vi "WSVCAP SHL FPGA LL I2C Procedure - Send Data Byte.vi"(0 "Procedure Step":T1, 1 "Wait Ticks Remaining":u32, 5 "I2C Wait Ticks":u32, 7 "Write Bits Remaining":u8, 11 "error in (no error)":errorcluster, 13 "Socket Mask":u32 format="%06x", 14 "UUT (0/1)":u8) -> (3 "Wait Ticks Remaining Out":u32, 4 "Procedure Step Out":T1, 8 "Write Bits Remaining Out":u8, 10 "Finished":bool, 15 "error out":errorcluster)   [LabVIEW 2017]
uses:
  Type Defs/WSVCAP SHL Procedure Step Enum.ctl
  Type Defs/WSVCAP SHL FIFO Operation Enum.ctl
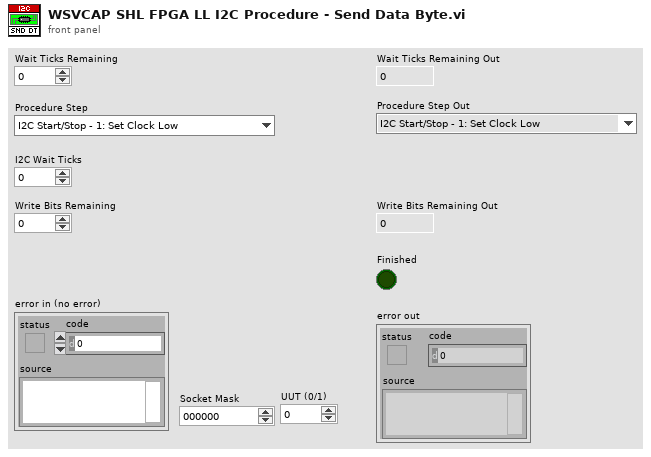
[diagram p1: front panel]
types:
  T1 = typedef "WSVCAP SHL Procedure Step Enum.ctl" = enum16{"I2C Start/Stop - 1: Set Clock Low", "I2C Start/Stop - 2: Wait", "I2C Start/Stop - 3: Set Data I", "I2C Start/Stop - 4: Wait", "I2C Start/Stop - 5: Set Clock High", "I2C Start/Stop - 6: Wait", "I2C Start/Stop - 7: Set Data II", "I2C Start/Stop - 8: Wait", "I2C Start/Stop - 9: Set Clock Low", "I2C Start/Stop - 10: Wait", "I2C Read ACK - 1: Set Clock High", "I2C Read ACK - 2: Wait", "I2C Read ACK - 3: Read ACK Bit", "I2C Read ACK - 4: Wait", "I2C Read ACK - 5: Set Clock Low", "I2C Read ACK - 6: Wait", "I2C Write ACK - 1: Write ACK Bit", "I2C Write ACK - 2: Wait", "I2C Write ACK - 3: Set Clock High", "I2C Write ACK - 4: Wait", "I2C Write ACK - 5: Set Clock Low", "I2C Write ACK - 6: Wait", "I2C Write ACK - 7: Set Data Low", "I2C Send Add - 1: Reset Bits Remaining", "I2C Send Add - 2: Set Data Bit", "I2C Send Add - 3: Wait", "I2C Send Add - 4: Set Clock High", "I2C Send Add - 5: Wait", "I2C Send Add - 6: Set Clock Low", "I2C Send Add - 7: Wait", "I2C Send Add - 8: Check Bits Remaining", "I2C Send Data - 1: Reset Bits Remaining", "I2C Send Data - 2: Load Write Bit from FIFO", "I2C Send Data - 3: Set Data Bit", "I2C Send Data - 4: Wait", "I2C Send Data - 5: Set Clock High", "I2C Send Data - 6: Wait", "I2C Send Data - 7: Set Clock Low", "I2C Send Data - 8: Wait", "I2C Send Data - 9: Check Bits Remaining", "I2C Receive Data - 1: Reset Bits Remaining", "I2C Receive Data - 2: Wait", "I2C Receive Data - 3: Set Clock High", "I2C Receive Data - 4: Wait", "I2C Receive Data - 5: Read Data Bit", "I2C Receive Data - 6: Wait", "I2C Receive Data - 7: Set Clock Low", "I2C Receive Data - 8: Wait", "I2C Receive Data - 9: Check Bits Remaining", "RFFE Send SSC - 1:Set Low", "RFFE Send SSC - 2:Wait", "RFFE Send SSC - 3:Set SDA High", "RFFE Send SSC - 4:Wait", "RFFE Send SSC - 5:Set SDA Low", "RFFE Send SSC - 6:Wait", "RFFE Send Data - 1:Set SCL High", "RFFE Send Data - 2:Wait", "RFFE Send Data - 3:Set SCL Low", "RFFE Send Data - 4:Wait", "RFFE Send Data - 5:Set SCL High (P)", "RFFE Send Data - 6:Wait", "RFFE Send Data - 7:Set SCL Low (P)", "RFFE Send Data - 8:Wait", "RFFE Send Data - 9:Set SCL High (BP)", "RFFE Send Data - 10:Wait", "RFFE Send Data - 11:Set SCL Low (BP)", "RFFE Send Data - 12:Wait", "RFFE Receive Data - 1:Set SCL High", "RFFE Receive Data - 2:Wait", "RFFE Receive Data - 3:Set SCL Low", "RFFE Receive Data - 4:Wait", "RFFE Receive Data - 5:Set SCL High (BP)", "RFFE Receive Data - 6:Wait", "RFFE Receive Data - 7:Set SCL Low (BP)", "RFFE Receive Data - 8:Wait", "RFFE Wait CMD Delay - 1:Wait", "RFFE Clear Lines - 1:Clear", "SRL Write Data - 1:Set SYNC High", "SRL Write Data - 2:Wait SYNC Delay", "SRL Write Data - 3:Set SYNC Low", "SRL Write Data - 4:Set SCLK High", "SRL Write Data - 5:Wait", "SRL Write Data - 6:Set SCLK Low", "SRL Write Data - 7:Wait", "SRL Write Data - 8:Set SYNC High", "SRL Wait CMD Delay - 1:Wait", "SRL Clear Lines - 1:Clear"}
  T2 = typedef "WSVCAP SHL FIFO Operation Enum.ctl" = enum16{"Create FIFO/Memory", "Get Write FIFO Status", "Get Read FIFO Status", "Put Element in Write", "Put Element in Read", "Get Element from Write", "Get Element from Read"}
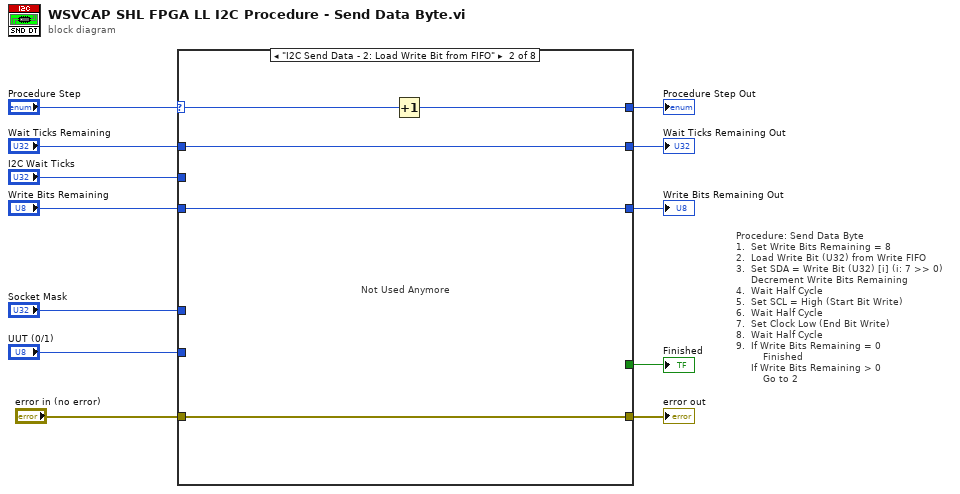
[diagram p0: block diagram]
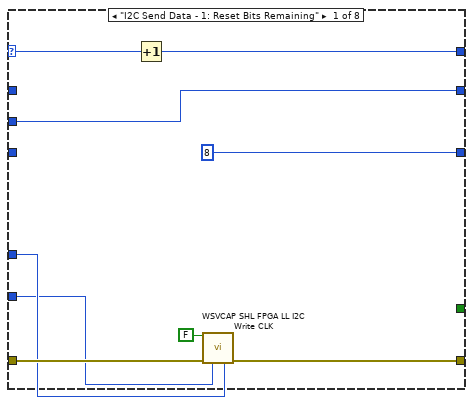
[diagram p2: hidden frame]
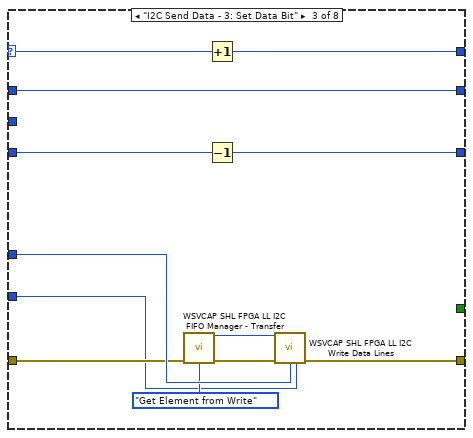
[diagram p3: hidden frame]
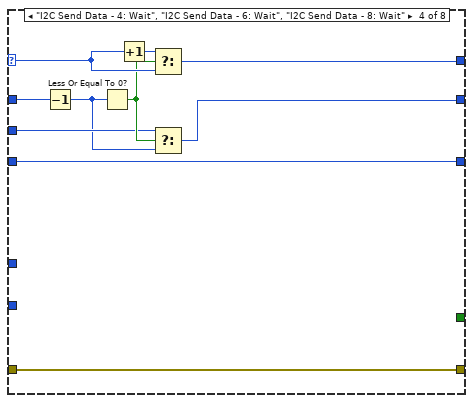
[diagram p4: hidden frame]
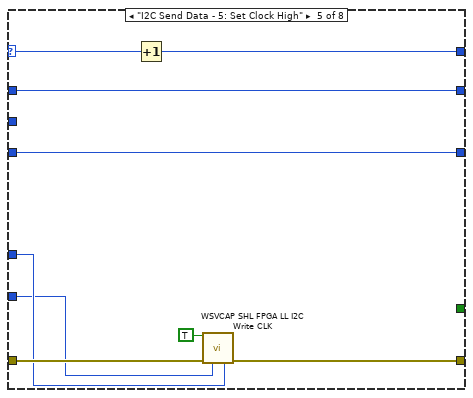
[diagram p5: hidden frame]
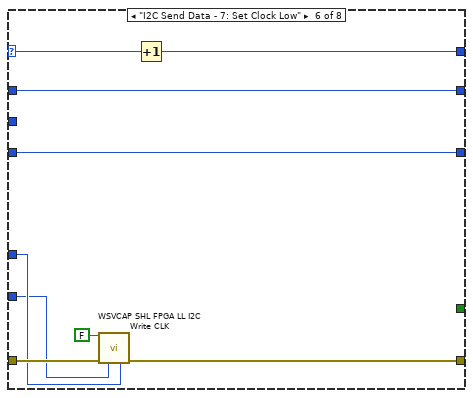
[diagram p6: hidden frame]
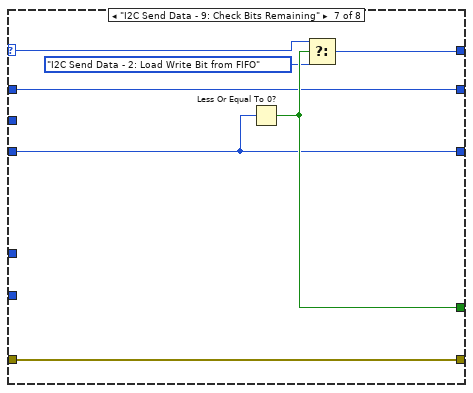
[diagram p7: hidden frame]
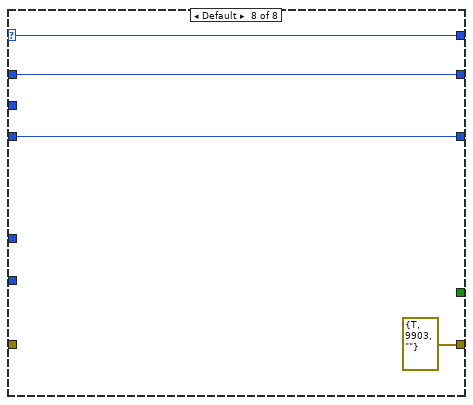
[diagram p8: hidden frame]
diagram:
  # "Procedure: Send Data Byte\n1.  Set Write Bits Remaining = 8\n2.  Load Write Bit (U32) from Write FIFO\n3.  Set SDA = Write Bit (U32) [i] (i: 7 >> 0)\n     Decrement Write Bits Remaining\n4.  Wait Half Cycle\n5.  Set SCL = High (Start Bit Write)\n6.  Wait Half Cycle\n7.  Set Clock Low (End Bit Write)\n8.  Wait Half Cycle\n9.  If Write Bits Remaining = 0\n         Finished\n     If Write Bits Remaining > 0\n         Go to 2"
  n1 = case shown="\"I2C Send Data - 2: Load Write Bit from FIFO\"" "Procedure Step" {
    selector: "Procedure Step" -> [w18 w26 w37 w47 w55 w63 w68 w76]
    tunnel: [w20 w22 w38 w45 w56 w65 w73 errorcluster {"status"=TRUE, "code"=9903, "source"=""} ("error IO")] -> w11
    tunnel: "error in (no error)" -> [w21 w22 w33 w45 w57 w66 w73 _]
    tunnel: "Wait Ticks Remaining" -> [_ w24 w28 w48 w51 w60 w67 w75]
    tunnel: "I2C Wait Ticks" -> [w16 _ _ w43 _ _ _ _]
    tunnel: "Write Bits Remaining" -> [_ w23 w36 w39 w50 w59 w69 w74]
    tunnel: [_ _ _ _ _ _ w72 _] -> w10
    tunnel: "Socket Mask" -> [w17 _ w35 _ w53 w62 _ _]
    tunnel: [w16 w24 w28 w41 w51 w60 w67 w75] -> w4
    tunnel: [u8 8 ("Write Bits Remaining") w23 w29 w39 w50 w59 w69 w74] -> w3
    tunnel: [w14 w25 w30 w40 w52 w61 w70 w76] -> w2
    tunnel: "UUT (0/1)" -> [w13 _ w27 _ w49 w58 _ _]
    frame "I2C Send Data - 1: Reset Bits Remaining" {
      n2 = Increment(x=w18) -> (x+1=w14:T1)
      n3 = call "WSVCAP SHL FPGA LL I2C Write CLK.vi"("Bit In"=FALSE, "error in (no error)"=w21, "UUT Set (0/1 (Legacy)"=w13, "Socket Mask"=w17) -> ("error out"=w20:errorcluster)  [unwired: 11 in]
    }
    frame "I2C Send Data - 2: Load Write Bit from FIFO" {
      # "Not Used Anymore"
      n4 = Increment(x=w26) -> (x+1=w25:T1)
    }
    frame "I2C Send Data - 3: Set Data Bit" {
      n5 = call "WSVCAP SHL FPGA LL I2C FIFO Manager - Transfer.vi"("error in (no error)"=w33, "Operation"=WSVCAP_SHL_FIFO_Operation_Enum."Get Element from Write") -> ("Data Out"=w31:u64, "error out"=w32:errorcluster)  [unwired: 11 in, 1 out]
      n6 = Increment(x=w37) -> (x+1=w30:T1)
      n7 = Decrement(x=w36) -> (x-1=w29:u8)
      n8 = call "WSVCAP SHL FPGA LL I2C Write Data Lines.vi"("Write Bit (U64)"=w31, "error in (no error)"=w32, "Socket Mask"=w35, "UUT Set (0/1) (Legacy)"=w27) -> ("error out"=w38:errorcluster)  [unwired: 11 in]
    }
    frame "I2C Send Data - 4: Wait", "I2C Send Data - 6: Wait", "I2C Send Data - 8: Wait" {
      n9 = Decrement(x=w48) -> (x-1=w42:u32)
      n10 = Less Or Equal To 0?(x=w42) -> (x <= 0?=w44:bool)
      n11 = Increment(x=w47) -> (x+1=w46:T1)
      n12 = Select(t=w46, s=w44, f=w47) -> (s? t:f=w40:T1)
      n13 = Select(t=w43, s=w44, f=w42) -> (s? t:f=w41:u32)
    }
    frame "I2C Send Data - 5: Set Clock High" {
      n14 = Increment(x=w55) -> (x+1=w52:T1)
      n15 = call "WSVCAP SHL FPGA LL I2C Write CLK.vi"("Bit In"=TRUE, "error in (no error)"=w57, "UUT Set (0/1 (Legacy)"=w49, "Socket Mask"=w53) -> ("error out"=w56:errorcluster)  [unwired: 11 in]
    }
    frame "I2C Send Data - 7: Set Clock Low" {
      n16 = call "WSVCAP SHL FPGA LL I2C Write CLK.vi"("Bit In"=FALSE, "error in (no error)"=w66, "UUT Set (0/1 (Legacy)"=w58, "Socket Mask"=w62) -> ("error out"=w65:errorcluster)  [unwired: 11 in]
      n17 = Increment(x=w63) -> (x+1=w61:T1)
    }
    frame "I2C Send Data - 9: Check Bits Remaining" {
      n18 = Less Or Equal To 0?(x=w69) -> (x <= 0?=w72:bool)
      n19 = Select(t=w68, s=w72, f=WSVCAP_SHL_Procedure_Step_Enum."I2C Send Data - 2: Load Write Bit from FIFO" ("Procedure Step")) -> (s? t:f=w70:T1)
    }
    frame Default {
    }
  }
  "error out" <- w11
  "Finished" <- w10
  "Procedure Step Out" <- w2
  "Wait Ticks Remaining Out" <- w4
  "Write Bits Remaining Out" <- w3
